vi "depth_camera.vi"(0 "Camera configuration":string="{\n     \"type\": \"DepthCamera\",\n      \"listen_port\": 8014,\n      \"location\": {\n       \"x\": 0.0,\n       \"y\": 0.0,\n       \"z\": 250.0\n     },\n     \"rotation\": {\n       \"pitch\": 0.0,\n       \"yaw\": 0.0,\n       \"roll\": 0.0\n     },\n     \"stream_dimensions\": {\n       \"x\": 512.0,\n       \"y\": 512.0\n     },\n    \"ray_tracing\":{\n        \"enable_ray_tracing\": false\n     },\n    \"dynamic_range\": 1.0,\n\t    \"fov\": 60.0,\n     \"camera_matrix\": [\n          [433.0, 0.0,   256.0],\n          [0.0,   433.0, 256.0],\n          [0.0,   0.0,   1.0]\n      ],\t\n\t    \"min_shutter\": 0.0005,\n\t    \"max_shutter\": 0.0014,\n     \"motion_blur_bias\": 0.1,\n     \"white_balance\": 0.0,\n     \"white_balance_temp_offset\": 0,\n     \"exposure_compensation\": -1.0,\n     \"image_noise_bias\": 0.05,\n     \"annotation\": {\n      \"include_annotation\": false,\n      \"desired_tags\": [\n        \"traffic_sign\", \"vehicle\"\n      ],\n      \"far_plane\": 10000.0,\n      \"include_tags\": true,\n      \"include_obb\": false,\n      \"cull_partial_frame\":false,\n      \"debug_draw\":false\n    },\n    \"max_distance\":50000.0,\n    \"channels\": \"gray\",\n    \"channel_depth\":4\n }", 3 "error in":errorcluster) -> (4 "Camera configuration":string, 6 "Image":picture, 7 "Raw data":sgl[](array[numeric]), 8 "Annotation":string, 9 "error out":errorcluster)   [LabVIEW 2019]
doc: "Configures and reads the data stream for a Depth Camera sensor and outputs a picture of the specified size on the Camera configuration."
uses:
  controls/Header.ctl
  tools/simx_common.vi
panel:
  in  "Distance (meters)":sgl[unit](slide)=46.464645 scale=0.0..100.0
  out "Header":T1 {"game_time" format="%_10g"}
  in  "Show Annotation":bool
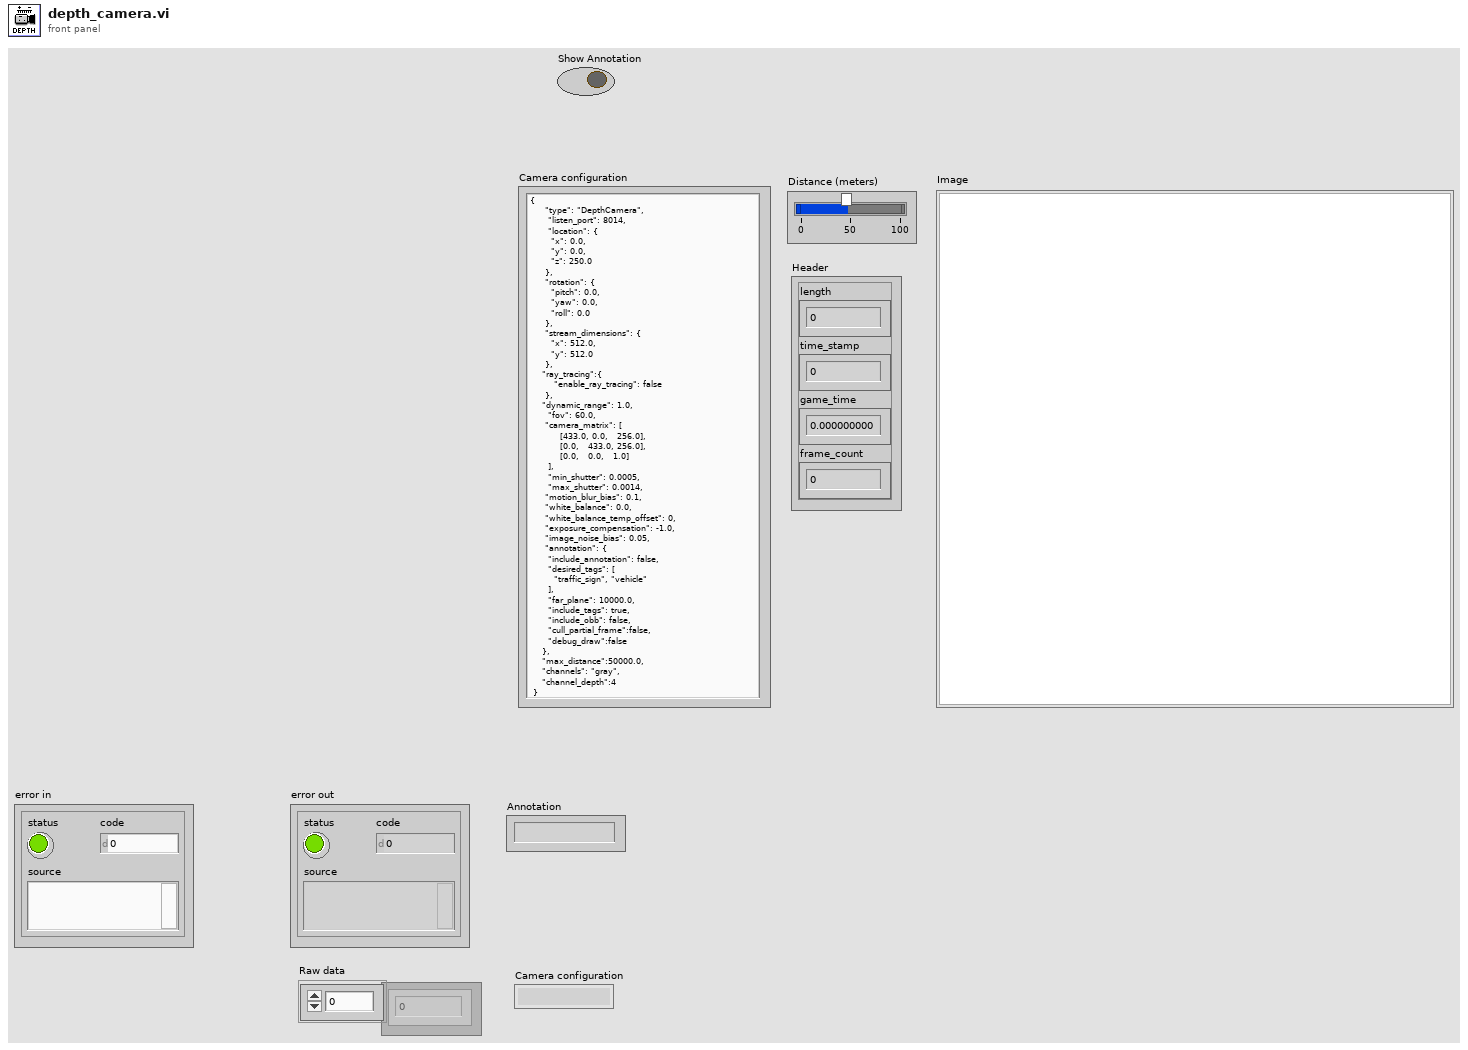
[diagram p1: front panel]
types:
  T1 = typedef "Header.ctl" = cluster{"length":u32, "time_stamp":u32, "game_time":sgl, "frame_count":u32}
  T2 = typedef "simx_connection.ctl" = cluster{"Config":T3, "Connections":T6, "Map":cluster{"lanes":cluster{"x":dbl[], "y":dbl[], "z":dbl[]}, "StartPosition":cluster{"start_points":T7, "StartRotation":dbl[], "StartLocation":dbl[]}, "Draw Map Size":T8, "DrawArea":cluster{"min_Y":dbl, "min_X":dbl, "Scale X":dbl, "Scale Y":dbl}, "Map":picture, "Map Geojson":string}}
  T3 = typedef "config.ctl" = cluster{"Trajectory":T4, "Weather":T5}
  T4 = typedef "trajectory.ctl" = cluster{"Number of frames":i32, "Frame number":i32, "Trajectory":string}
  T5 = typedef "weather.ctl" = cluster{"id":string}
  T6 = typedef "connections.ctl" = cluster{"Simulator Connection":refnum<k5>, "server_ip":string, "Port":i32, "Sensor connections":refnum<k5>[]}
  T7 = typedef "start_points.ctl" = cluster{"locations":dbl[][], "rotations":dbl[][], "type":string[]}
  T8 = typedef "LVBoundsTypeDef.ctl" = cluster{"Width":u32, "Height":u32}
  T9 = typedef "sensor_sample.ctl" = cluster{"Header":T1, "data out":string}
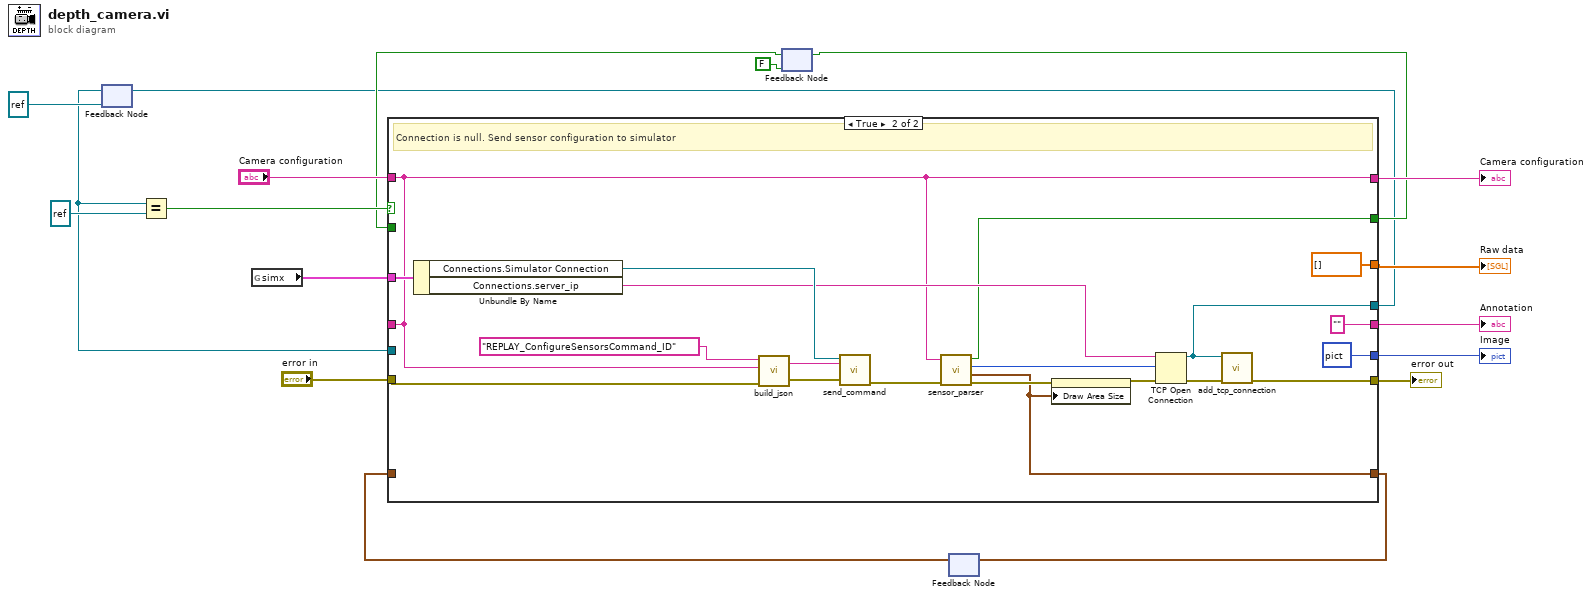
[diagram p0: block diagram]
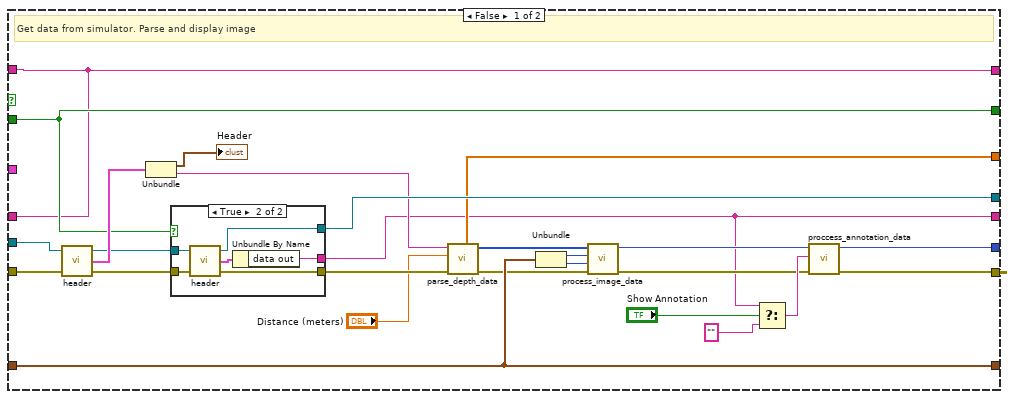
[diagram p2: hidden frame]
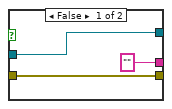
[diagram p3: hidden frame]
diagram:
  n1 = feedback #1(refnum<k5> refnum ("camera_connection")) -> (w5:refnum<k5>)
  n2 = Equal?(x=w5, y=refnum<k5> refnum ("null connection")) -> (x = y?=w7:bool)
  n3 = global read "simx_common.vi" "simx"() -> (w9:T2)
  n4 = feedback #2(FALSE) -> (w6:bool)
  n5 = feedback #3() -> (w10:cluster{"x dimension":i32, "y dimension":i32})  [unwired: 1 in]
  n6 = case shown="True" w7 {
    tunnel: [w39 w56] -> w12
    tunnel: [w27 w55] -> _
    tunnel: [w32 w58] -> w1
    tunnel: w5 -> [w43 _]
    tunnel: "error in" -> [w42 w65]
    tunnel: w10 -> [w41 _]
    tunnel: [w38 picture data[5B] ("new picture")] -> w3
    tunnel: [w41 w62] -> w11
    tunnel: [w27 w55] -> w15
    tunnel: [w40 w61] -> w8
    tunnel: w6 -> [w40 _]
    tunnel: [w19 "" ("data out")] -> w2
    tunnel: w9 -> [_ w59]
    tunnel: "Camera configuration" -> [w27 w55]
    tunnel: [w21 sgl[] [] ("Raw data")] -> w4
    frame False {
      # "Get data from simulator. Parse and display image"
      n7 = call "header.vi"("error in"=w42, "TCP Network Connection in"=w43) -> ("error out"=w26:errorcluster, "Sensor sample"=w44:T9, "TCP Network Connection out"=w36:refnum<k5>)  [unwired: 1 in]
      n8 = Unbundle(w44) -> ("Header"=→"Header":T1, "data out"=w23:string)
      n9 = case shown="True" w40 {
        tunnel: w36 -> [w47 w53]
        tunnel: [w47 w52] -> w32
        tunnel: w26 -> [w46 w51]
        tunnel: [w46 w49] -> w25
        tunnel: ["" ("data out") w48] -> w19
        frame False {
        }
        frame True {
          n10 = call "header.vi"("error in"=w51, "TCP Network Connection in"=w53) -> ("error out"=w49:errorcluster, "Sensor sample"=w50:T9, "TCP Network Connection out"=w52:refnum<k5>)  [unwired: 1 in]
          n11 = Unbundle By Name(w50) -> ("data out"=w48:string)
        }
      }
      n12 = call "parse_depth_data.vi"("error in"=w25, "Distance (meters)"="Distance (meters)", "Data"=w23) -> ("error out"=w24:errorcluster, "Normalized data"=w20:u8[], "Raw data"=w21:sgl[])  [unwired: 2 in]
      n13 = Unbundle(w41) -> ("x dimension"=w30:i32, "y dimension"=w29:i32)
      n14 = call "process_image_data.vi"("error in"=w24, "y"=w29, "x"=w30, "Raw data"=w20) -> ("error out"=w31:errorcluster, "Image"=w28:picture)  [unwired: 4 in]
      n15 = Select(t=w19, s="Show Annotation", f="") -> (s? t:f=w33:string)
      n16 = call "proccess_annotation_data.vi"("error in"=w31, "Annotation Data"=w33, "Image in"=w28) -> ("error out"=w39:errorcluster, "Image out"=w38:picture)  [unwired: 2 in, 1 out]
    }
    frame True {
      # "Connection is null. Send sensor configuration to simulator"
      n17 = Unbundle By Name(w59) -> ("Connections.Simulator Connection"=w68:refnum<k5>, "Connections.server_ip"=w66:string)
      n18 = call "build_json.vi"("error in"=w65, "Message"=w55, "Command_ID"="REPLAY_ConfigureSensorsCommand_ID") -> ("error out"=w71:errorcluster, "JSON Out"=w72:string)  [unwired: 1 in]
      n19 = call "send_command.vi"("error in"=w71, "JSON Command"=w72, "TCP Network Connection in"=w68) -> ("error out"=w64:errorcluster)  [unwired: 1 in, 3 out]
      n20 = call "sensor_parser.vi"("Sensor configuration"=w55, "error in"=w64) -> ("include_annotation"=w61:bool, "Port out"=w60:u16, "Stream dimensions"=w62:cluster{"x dimension":i32, "y dimension":i32}, "error out"=w63:errorcluster)  [unwired: 1 in]
      n21 = property on="Image" class="Pict"(error in=w63, "Draw Area Size"=w62) -> (error out=w67:errorcluster)  [unwired: 1 in, 1 out]
      n22 = TCP Open Connection(address=w66, remote port or service name=w60, error in (no error)=w67) -> (connection ID=w58:refnum<k5>, error out=w57:errorcluster)  [unwired: 2 in]
      n23 = call "add_tcp_connection.vi"("error in"=w57, "Sensor connection"=w58) -> ("error out"=w56:errorcluster)  [unwired: 5 in]
    }
  }
  "error out" <- w12
  "Raw data" <- w4
  "Camera configuration" <- w15
  "Image" <- w3
  "Annotation" <- w2
  n24 = feedback-in #1(w1) -> ()
  n25 = feedback-in #2(w8) -> ()
  n26 = feedback-in #3(w11) -> ()
